vi "Processed_To_Raw_Bytes.vi"(6 "Processed Bytes":u8[](array[numeric])=[0, 0, 0, 0, 0, 0, 0, 0, 0]) -> (0 "Packet Type":T2, 1 "Checksum":bool, 2 "Node ID":u8, 3 "Raw Bytes":u8[](array[numeric]), 4 "Priority":T1)   [LabVIEW 2017]
uses:
  Controls/Packet/Packet_Type.ctl
  Controls/Packet/Packet_Priority.ctl
panel:
  out "Frame ID":u8
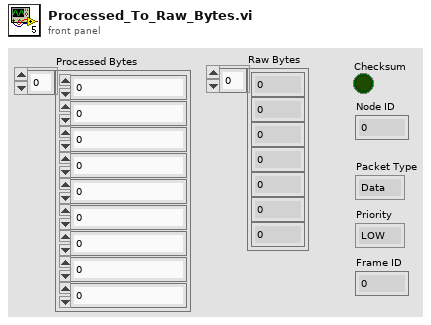
[diagram p1: front panel]
types:
  T1 = typedef "Packet_Priority.ctl" = enum16{"LOW", "HIGH"}
  T2 = typedef "Packet_Type.ctl" = enum16{"Data", "Connection Management", "Remote Request", "Error/Status"}
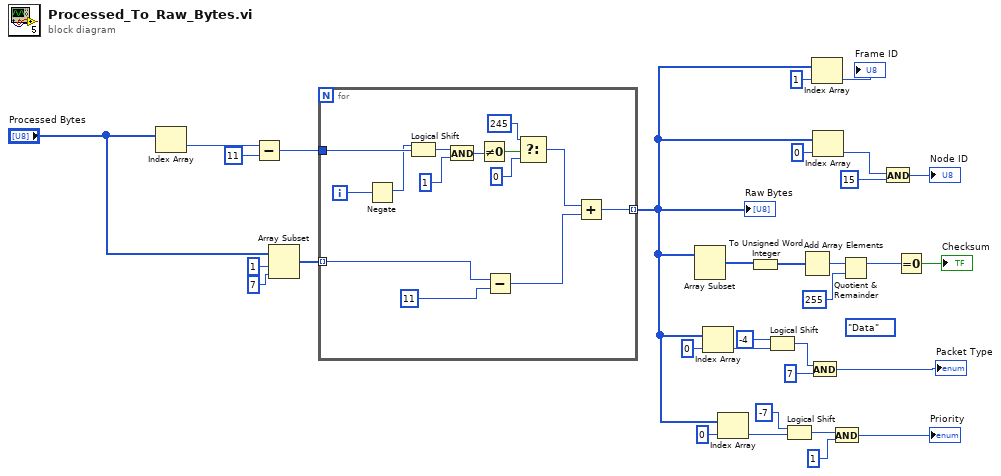
[diagram p0: block diagram]
diagram:
  (unwired) Packet_Type."Data" ("Packet type")
  n1 = Index Array(array="Processed Bytes") -> (element=w32:u8)  [unwired: 1 in]
  n2 = Subtract(x=w32, y=u8 11) -> (x-y=w20:u8)
  n3 = Array Subset(array="Processed Bytes", index=1, length=7) -> (w28:u8[])
  n4 = for {
    tunnel: w28 -> [w46] mode=indexing
    tunnel: [w40] -> w3 mode=indexing
    tunnel: w20 -> [w39]
    i -> [w38]
    n5 = Negate(x=w38) -> (-x=w37:i32)
    n6 = Logical Shift(y=w37, x=w39) -> (x << y=w36:u8)
    n7 = And(x=w36, y=u8 1) -> (x .and. y?=w34:u8)
    n8 = Not Equal To 0?(x=w34) -> (x != 0?=w33:bool)
    n9 = Subtract(x=w46, y=u8 11) -> (x-y=w41:u8)
    n10 = Select(t=u8 245 ("y"), s=w33, f=u8 0) -> (s? t:f=w42:u8)
    n11 = Add(x=w42, y=w41) -> (x+y=w40:u8)
  }
  "Raw Bytes" <- w3
  n12 = Array Subset(array=w3) -> (w26:u8[])  [unwired: 2 in]
  n13 = Index Array(array=w3, index=0) -> (element=w14:u8)
  n14 = Index Array(array=w3, index=0) -> (element=w9:u8)
  n15 = To Unsigned Word Integer(number=w26) -> (unsigned 16bit integer=w25:u16[])
  n16 = Logical Shift(y=i16 -4, x=w14) -> (x << y=w12:u8)
  n17 = Logical Shift(y=i16 -7, x=w9) -> (x << y=w7:u8)
  n18 = Add Array Elements(numeric array=w25) -> (sum=w24:u16)
  n19 = And(x=w12, y=u8 7) -> (x .and. y?=→"Packet Type":u8)
  n20 = Index Array(array=w3, index=1) -> (element=→"Frame ID":u8)
  n21 = Index Array(array=w3, index=0) -> (element=w18:u8)
  n22 = And(x=w7, y=u8 1) -> (x .and. y?=→"Priority":u8)
  n23 = Quotient & Remainder(x=w24, y=u16 255) -> (x-y*floor(x/y)=w22:u16)  [unwired: 1 out]
  n24 = And(x=w18, y=u8 15) -> (x .and. y?=→"Node ID":u8)
  n25 = Equal To 0?(x=w22) -> (x = 0?=→"Checksum":bool)
